vi "H-bridge.vi"(10 "Mode":T1(radio)) -> (2 "output relays":T2)   [LabVIEW 2009]
doc: "This VI is intended for a relay H-bridge motor controller. (four single-directional relays)"
panel:
  # "This VI is intended for a relay H-bridge\n(with 4 one-directional relays)\nHere's an example wiring daigram:"
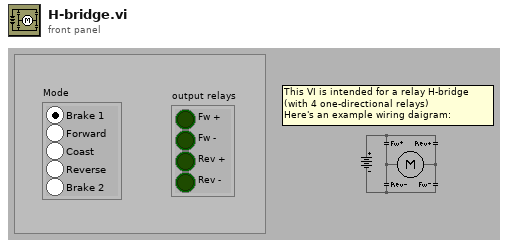
[diagram p1: front panel]
types:
  T1 = enum32{"Brake 1", "Forward", "Coast", "Reverse", "Brake 2"}
  T2 = cluster{"Fw +":bool, "Fw -":bool, "Rev +":bool, "Rev -":bool}
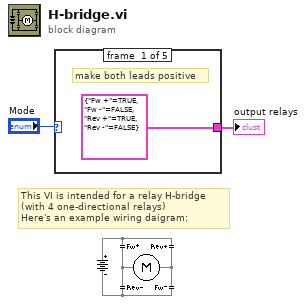
[diagram p0: block diagram]
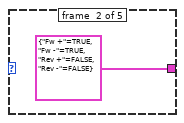
[diagram p2: hidden frame]
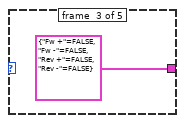
[diagram p3: hidden frame]
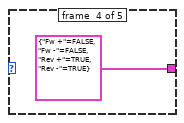
[diagram p4: hidden frame]
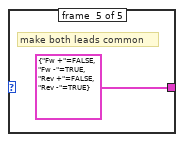
[diagram p5: hidden frame]
diagram:
  # "This VI is intended for a relay H-bridge\n(with 4 one-directional relays)\nHere's an example wiring daigram:"
  n1 = case shown="\"Forward\"" "Mode" {
    tunnel: [T2 {"Fw +"=TRUE, "Fw -"=FALSE, "Rev +"=TRUE, "Rev -"=FALSE} ("output relays") T2 {"Fw +"=TRUE, "Fw -"=TRUE, "Rev +"=FALSE, "Rev -"=FALSE} ("output relays") T2 {"Fw +"=FALSE, "Fw -"=FALSE, "Rev +"=FALSE, "Rev -"=FALSE} ("output relays") T2 {"Fw +"=FALSE, "Fw -"=FALSE, "Rev +"=TRUE, "Rev -"=TRUE} ("output relays") T2 {"Fw +"=FALSE, "Fw -"=TRUE, "Rev +"=FALSE, "Rev -"=TRUE} ("output relays")] -> w1
    frame #0 {
      # "make both leads positive"
    }
    frame #1 {
    }
    frame #2 {
    }
    frame #3 {
    }
    frame #4 {
      # "make both leads common"
    }
  }
  "output relays" <- w1
